vi "Fetch_Destination.vi"(8 "error in (no error)":errorcluster, 10 "destTag":string, 11 "Installer in":refnum<class "Installer.lvclass">) -> (0 "error out":errorcluster, 2 "index":i32, 3 "IB_Destination.lvclass":refnum<class "IB_Destination.lvclass">)   [LabVIEW 2020, in "Installer.lvclass"]
uses:
  <vilib>/AppBuilder/IB_Classes/Installer/Installer.lvclass
  <vilib>/AppBuilder/IB_Classes/Installer/Installer.lvclass/Installer.ctl
  <vilib>/AppBuilder/IB_Classes/Destination/IB_Destination.lvclass
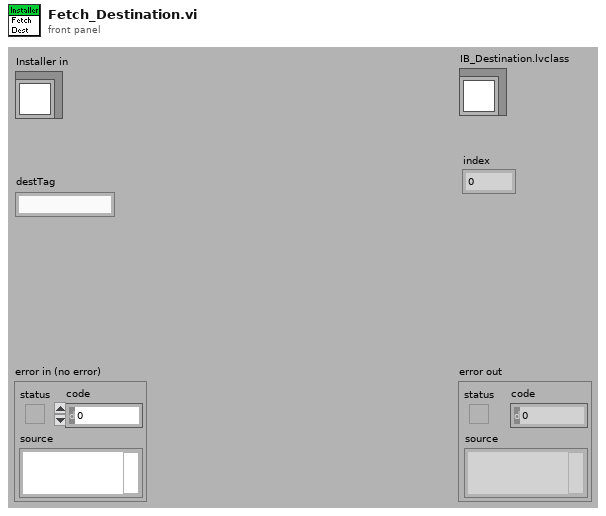
[diagram p1: front panel]
types:
  T1 = typedef "IB_Destination.ctl" = cluster{"name":string, "unlock":bool, "parentTag":string, "destTag":string, "eng_installPath":string}
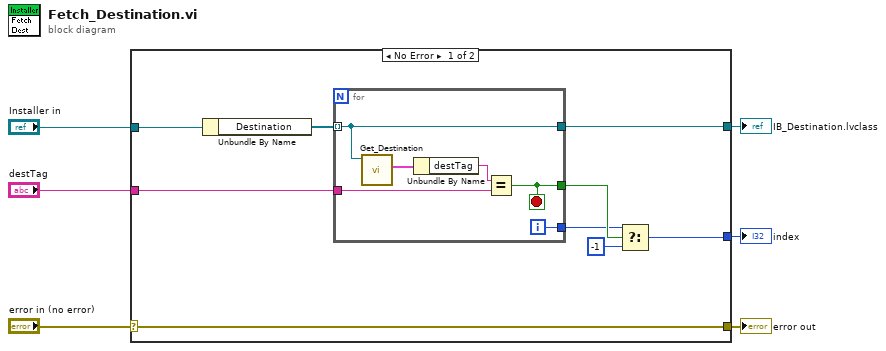
[diagram p0: block diagram]
diagram:
  n1 = case shown="No Error" "error in (no error)" {
    selector: "error in (no error)" -> [w15 w22]
    tunnel: [w15 w22] -> w5
    tunnel: "Installer in" -> [w14 _]
    tunnel: "destTag" -> [w12 _]
    tunnel: [w11 _] -> w2
    tunnel: [w7 _] -> w1
    frame No Error {
      n2 = Unbundle By Name(w14) -> ("Destination"=w13:refnum<class "IB_Destination.lvclass">[])
      n3 = for {
        tunnel: w13 -> [w18] mode=indexing
        tunnel: w12 -> [w19]
        tunnel: [w18] -> w11
        tunnel: [w17] -> w10
        tunnel: [w16] -> w9
        i -> [w16]
        stop <- w17 stop-if-true
        n4 = call <vilib>:"Get_Destination.vi"("IB_Destination in"=w18) -> ("data"=w21:T1)  [unwired: 8 in, 2 out]
        n5 = Unbundle By Name(w21) -> ("destTag"=w20:string)
        n6 = Equal?(x=w20, y=w19) -> (x = y?=w17:bool)
      }
      n7 = Select(t=w9, s=w10, f=-1) -> (s? t:f=w7:i32)
    }
    frame Error {
    }
  }
  "error out" <- w5
  "IB_Destination.lvclass" <- w2
  "index" <- w1
